vi "Stop Core.vi"(10 "final error code":i32, 11 "PLCHandler in":refnum<class "PLCHandler.lvclass">) -> (3 "PLCHandler out":refnum<class "PLCHandler.lvclass">)   [LabVIEW 2021, in "PLCHandler.lvlib" / "PLCHandler.lvclass"]
doc: "(<B>Filename</B>: Actor Framework.lvlib:Actor.lvclass:Stop Core.vi)\n\nDefines what the actor does before it stops. Use the <B>final error code</B> input to determine whether the actor shut down in response to an error.\n\nBy default, this method does nothing. A descendant class may override it to define behavior, such as shutting down any processes the actor initiated in its override of the Actor Core method."
uses:
  PLCHandler.lvclass
  <vilib>/ActorFramework/Actor/Actor.lvclass
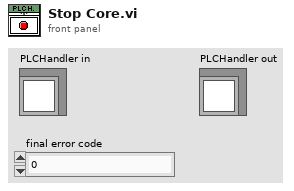
[diagram p1: front panel]
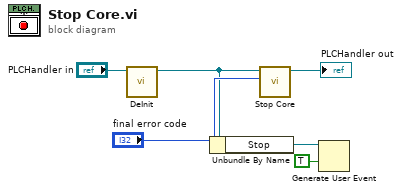
[diagram p0: block diagram]
diagram:
  n1 = call "DeInit.vi"("PLCHandler in"="PLCHandler in") -> ("PLCHandler out"=w3:refnum<class "PLCHandler.lvclass">)  [unwired: 9 in, 1 out]
  n2 = Unbundle By Name(w3) -> ("Stop"=w2:refnum<user-event>)
  n3 = call-parent "Stop Core.vi"("final error code"="final error code", "Actor in"=w3) -> ("Actor out"=→"PLCHandler out":refnum<class "PLCHandler.lvclass">)  [unwired: 9 in]
  n4 = Generate User Event(user event=w2, event data cluster=TRUE ("event data")) -> ()  [unwired: 2 in, 2 out]
